vi "RT Loop - Acquire camera_data_queue_test.vi"(8 "Boolean":bool, 11 "Message Queue":refnum<queue>) -> ()   [LabVIEW 2017]
uses:
  UI Error Handlers/support/Message Queue/Message Cluster.ctl
  <vilib>/vision/Image Controls.llb/IMAQ Image.ctl
  <vilib>/userdefined/High Color/IMAQdx.ctl
  <vilib>/vision/Avi.llb/IMAQ AVI2 Codec Path.ctl
  Globals/Global - All RT Loop Stop.vi
  Globals/Global - Configuration Options.vi
  <vilib>/vision/driver/NI_Vision_Acquisition_Software.lvlib
  UI Error Handlers/support/Message Queue/Message Queue.lvlib
panel:
  out "Cluster":cluster{"Image Out":T1, "AVI Path 2":path}
  out "AVI Path":path
  out "Acceleration Log Folder":path=path "/home/lvuser/Log/logfiles_deploy"
  out "Codec Names":string[](array[string])
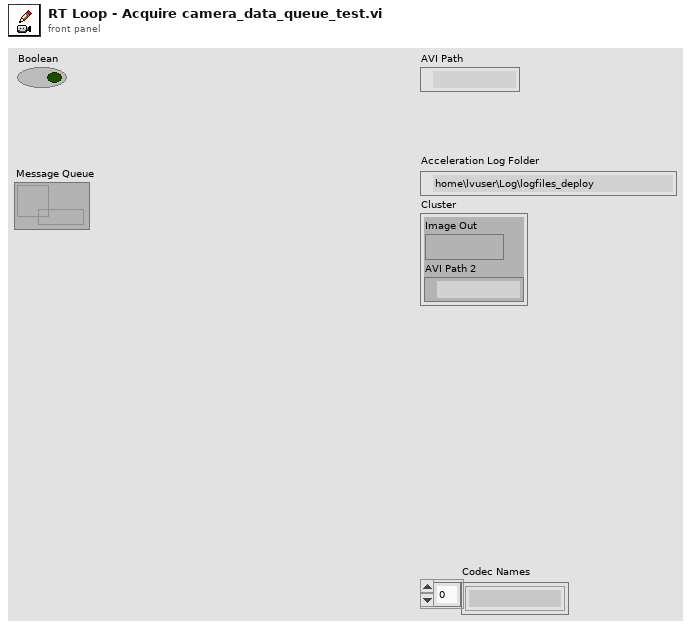
[diagram p1: front panel]
types:
  T1 = typedef "IMAQ Image.ctl" = refnum<image>
  T2 = typedef "IMAQdx.ctl" = refnum<k21>
  T3 = typedef "Image Type" = u32
  T4 = typedef "IMAQ AVI2 Codec Path.ctl" = u32
  T5 = cluster{"Tool data":cluster{"Number of teeth":sgl}, "Cutting data":cluster{"rpm":sgl}, "Limits":cluster{"Magnitude threshold":sgl, "Tolerance":sgl}, "G1 status":cluster{"G1 trigger":bool}}
  T6 = typedef "IMAQ AVI2 Refnum.ctl" = refnum<k20>
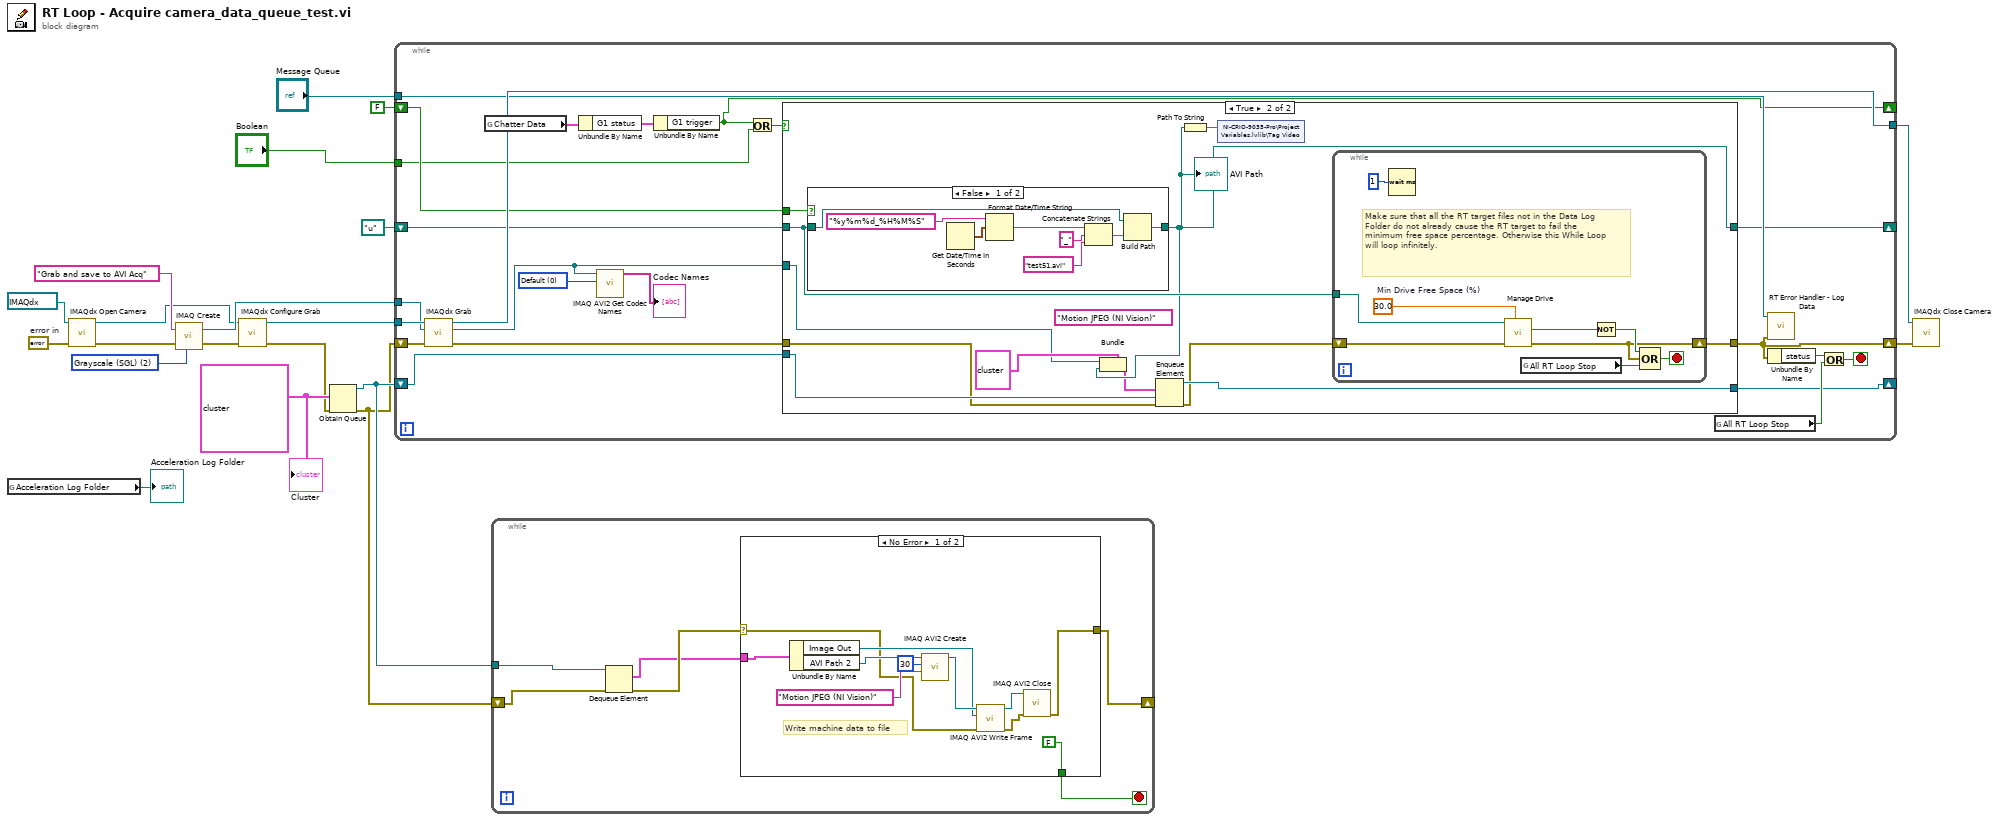
[diagram p0: block diagram]
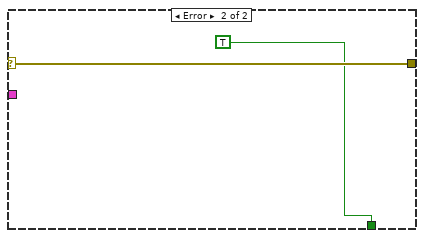
[diagram p2: hidden frame]
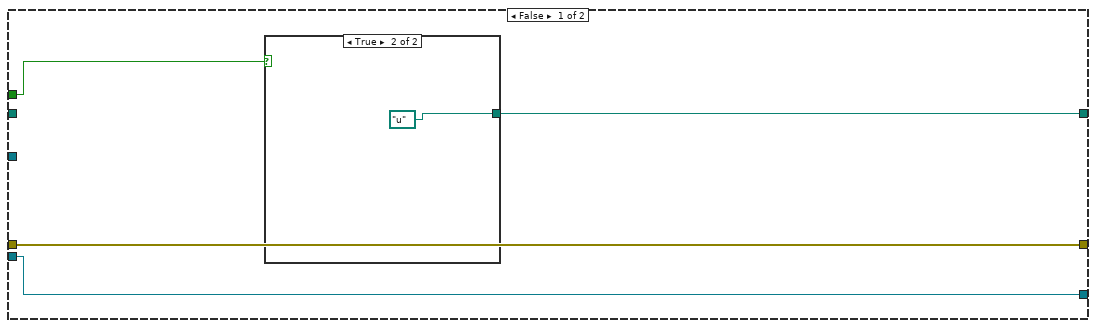
[diagram p3: hidden frame]
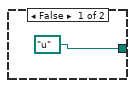
[diagram p4: hidden frame]
diagram:
  w4 = cluster{"Image Out":T1, "AVI Path 2":path} {"Image Out"=refnum, "AVI Path 2"=path ""}
  w17 = T3 2 items=["Grayscale (U8)", "Grayscale (I16)", "Grayscale (SGL)", "Complex (CSG)", "RGB (U32)", "HSL (U32)", "RGB (U64)", "Grayscale (U16)"] ("Image Type")
  w15 = errorcluster {"status"=FALSE, "code"=0, "source"=""}  # error in
  n1 = global read "Global - Configuration Options.vi" "Acceleration Log Folder"() -> (→"Acceleration Log Folder":path)
  n2 = call <vilib>:"IMAQdx Open Camera.vi"("error in"=w15, "Session In"=T2 "cam0") -> ("error out"=w18:errorcluster, "Session Out"=w13:T2)  [unwired: 8 in]
  n3 = call "IMAQ Create"("Image Name"="Grab and save to AVI Acq", "Image Type"=w17, "error in (no error)"=w18) -> ("New Image"=w20:T1, "error out"=w7:errorcluster)  [unwired: 2 in]
  n4 = call <vilib>:"IMAQdx Configure Grab.vi"("error in"=w7, "Session In"=w13) -> ("error out"=w3:errorcluster, "Session Out"=w19:T2)  [unwired: 8 in]
  n5 = Obtain Queue(element data type=w4, error in (no error)=w3) -> (queue out=w5:refnum<queue>, error out=w2:errorcluster)  [unwired: 3 in, 1 out]
  n6 = while {
    tunnel: w19 -> [w42]
    tunnel: w20 -> [w41]
    tunnel: [w40] -> w12
    tunnel: "Message Queue" -> [w32]
    shift-right: [w22] -> _
    shift-left: FALSE ("G1 trigger") -> [w28]
    shift-right: [w27] -> _
    shift-left: path "u:/" ("AVI Path") -> [w34]
    tunnel: "Boolean" -> [w26]
    shift-right: [w23] -> _
    shift-left: w5 -> [w24]
    shift-right: [w21] -> w1
    shift-left: w2 -> [w43]
    stop <- w38 stop-if-true
    w37 = T4 0 items=["Default", "System", "Built in Vision"] ("Codec Source")
    n7 = call <vilib>:"IMAQdx Grab.vi"("error in"=w43, "Image In"=w41, "Session In"=w42) -> ("error out"=w35:errorcluster, "Image Out"=w25:T1, "Session Out"=w40:T2)  [unwired: 5 in, 1 out]
    n8 = global read "Global - Configuration Options.vi" "Chatter Data"() -> (w31:T5)
    n9 = Unbundle By Name(w31) -> ("G1 status"=w30:cluster{"G1 trigger":bool})
    n10 = call "IMAQ AVI2 Get Codec Names"("Codec Source"=w37, "Image"=w25) -> ("Codec Names"=→"Codec Names":string[])  [unwired: 8 in, 1 out]
    n11 = Unbundle By Name(w30) -> ("G1 trigger"=w22:bool)
    n12 = Or(x=w22, y=w26) -> (x .or. y?=w29:bool)
    n13 = case shown="True" w29 {
      tunnel: w25 -> [_ w54]
      tunnel: w35 -> [w47 w50]
      tunnel: [w47 w61] -> w21
      tunnel: w34 -> [_ w60]
      tunnel: w28 -> [w46 w59]
      tunnel: [w45 w53] -> w27
      tunnel: w24 -> [w44 w57]
      tunnel: [w44 w56] -> w23
      frame False {
        n14 = case shown="True" w46 {
          tunnel: [path "u:/" ("AVI Path") path "u:/" ("AVI Path")] -> w45
          frame False {
          }
          frame True {
          }
        }
      }
      frame True {
        (unwired) "Motion JPEG (NI Vision)" ("Codec")
        n15 = case shown="False" w59 {
          tunnel: w60 -> [w63 w70]
          tunnel: [w62 w70] -> w53
          frame False {
            n16 = Get Date/Time In Seconds() -> (seconds since 1Jan1904=w65:timestamp)
            n17 = Format Date/Time String(time format string (%c)="%y%m%d_%H%M%S", seconds (now)=w65) -> (date/time string=w66:string)  [unwired: 1 out]
            n18 = Concatenate Strings(w66, "_" ("string"), "test51.avi" ("name or relative path")) -> (w69:string)
            n19 = Build Path(base path=w63, name or relative path=w69) -> (appended path=w62:path)
          }
          frame True {
          }
        }
        "AVI Path" <- w53
        n20 = Bundle(cluster=cluster{"Image Out":T1, "AVI Path 2":path} {"Image Out"=refnum, "AVI Path 2"=path ""} ("Cluster 2"), "Image Out"=w54, "AVI Path 2"=w53) -> (w52:cluster{"Image Out":T1, "AVI Path 2":path})
        n21 = Enqueue Element(queue=w57, element=w52, error in (no error)=w50) -> (queue out=w56:refnum<queue>, error out=w51:errorcluster)  [unwired: 1 in, 1 out]
        n22 = Path To String(path=w53) -> (string=w58:string)
        n23 = shared-variable "NI-CRIO-9035-Pro\\Project Variables.lvlib\\Tag Video"(w58) -> ()  [unwired: 1 in, 1 out]
        n24 = while {
          shift-right: [w74] -> w61
          shift-left: w51 -> [w75]
          tunnel: w60 -> [w72]
          stop <- w79 stop-if-true
          w73 = 30.0  # Min Drive Free Space (%)
          # "Make sure that all the RT target files not in the Data Log Folder do not already cause the RT target to fail the minimum free space percentage. Otherwise this While Loop will loop infinitely."
          n25 = Wait (ms)(milliseconds to wait=u32 1) -> ()  [unwired: 1 out]
          n26 = call "Manage Drive.vi"("Min Drive Free Space (%)"=w73, "error in"=w75, "Data Folder"=w72) -> ("error out"=w74:errorcluster, "Drive Space Below Limit"=w71:bool)  [unwired: 7 in]
          n27 = global read "Global - All RT Loop Stop.vi" "All RT Loop Stop"() -> (w76:bool)
          n28 = Not(x=w71) -> (.not. x?=w78:bool)
          n29 = Compound Arithmetic op=OR(w78, w74, w76) -> (w79:bool)
        }
      }
    }
    n30 = global read "Global - All RT Loop Stop.vi" "All RT Loop Stop"() -> (w33:bool)
    n31 = call "RT Error Handler - Log Data.vi"("error in (no error)"=w21, "Message Queue"=w32) -> ()  [unwired: 9 in, 1 out]
    n32 = Unbundle By Name(w21) -> ("status"=w39:bool)
    n33 = Or(x=w39, y=w33) -> (x .or. y?=w38:bool)
  }
  n34 = while {
    tunnel: w5 -> [w85]
    shift-right: [w81] -> _
    shift-left: w2 -> [w82]
    stop <- w80 stop-if-true
    n35 = Dequeue Element(queue=w85, error in (no error)=w82) -> (element=w83:cluster{"Image Out":T1, "AVI Path 2":path}, error out=w84:errorcluster)  [unwired: 1 in, 2 out]
    n36 = case shown="No Error" w84 {
      selector: w84 -> [w90 w98]
      tunnel: [w86 w98] -> w81
      tunnel: w83 -> [w96 _]
      tunnel: [FALSE TRUE] -> w80
      frame No Error {
        # "Write machine data to file"
        n37 = Unbundle By Name(w96) -> ("Image Out"=w91:T1, "AVI Path 2"=w95:path)
        n38 = call "IMAQ AVI2 Create"("Codec"="Motion JPEG (NI Vision)", "Frames Per Second"=u32 30, "AVI Path"=w95) -> ("AVI Refnum"=w92:T6)  [unwired: 7 in, 1 out]
        n39 = call "IMAQ AVI2 Write Frame"("error in (no error)"=w90, "Image"=w91, "AVI Refnum"=w92) -> ("error out"=w87:errorcluster, "AVI Refnum (duplicate)"=w88:T6)  [unwired: 6 in, 1 out]
        n40 = call "IMAQ AVI2 Close"("error in (no error)"=w87, "AVI Refnum"=w88) -> ("error out"=w86:errorcluster)  [unwired: 9 in]
      }
      frame Error {
      }
    }
  }
  n41 = call <vilib>:"IMAQdx Close Camera.vi"("error in"=w1, "Session In"=w12) -> ()  [unwired: 9 in, 1 out]
  "Cluster" <- w4
